vi "Compare.vi"(8 "error in":errorcluster, 10 "Actual":refnum<class "CANopen Response Message.lvclass">, 11 "Initiate Down-Upload Response Comparator in":refnum<class "Initiate Down-Upload Response Comparator.lvclass">) -> (0 "error out":errorcluster, 2 "Equal?":bool, 3 "Initiate Down-Upload Response Comparator out":refnum<class "Initiate Down-Upload Response Comparator.lvclass">)   [LabVIEW 2024, in "CANopen Master.lvlib" / "Initiate Down-Upload Response Comparator.lvclass"]
uses:
  Initiate Down-Upload Response Comparator.lvclass
  D:/git/CANopen-XNET/SDO Response Compare Strategy/SDO Response Compare Strategy.lvclass
  CANopen Response/CANopen Response Message.lvclass
  D:/git/CANopen-XNET/CANopen Message/CANopen Message.lvclass
  SDO Response Compare Strategy/SDO Response Compare Strategy.lvclass/SDO Response Compare Strategy.ctl
  CANopen Message/CANopen Message.lvclass/CANopen Message.ctl
  CANopen Message/CANopen Message.lvclass
  SDO Response Compare Strategy/SDO Response Compare Strategy.lvclass
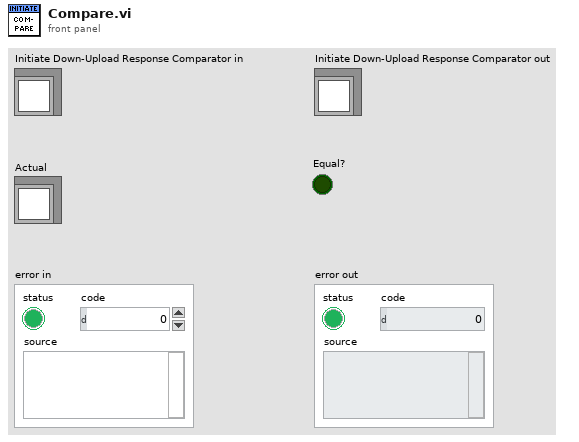
[diagram p1: front panel]
types:
  T1 = typedef "CANopen Master.lvlib/Multiplexor.ctl" = cluster{"Index":u16, "Sub-Index":u8}
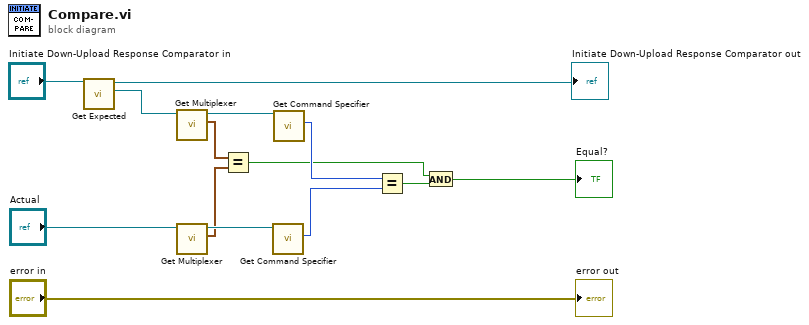
[diagram p0: block diagram]
diagram:
  n1 = call "Get Expected.vi"("SDO Response Compare Strategy in"="Initiate Down-Upload Response Comparator in") -> ("Expected Response Message"=w4:refnum<class "CANopen Response Message.lvclass">, "SDO Response Compare Strategy out"=→"Initiate Down-Upload Response Comparator out":refnum<class "Initiate Down-Upload Response Comparator.lvclass">)  [unwired: 9 in]
  n2 = call "Get Multiplexer.vi"("CANopen Message in"=w4) -> ("Multiplexer"=w9:T1, "CANopen Message out"=w11:refnum<class "CANopen Response Message.lvclass">)  [unwired: 9 in]
  n3 = call "Get Multiplexer.vi"("CANopen Message in"="Actual") -> ("Multiplexer"=w8:T1, "CANopen Message out"=w10:refnum<class "CANopen Response Message.lvclass">)  [unwired: 9 in]
  n4 = Equal?(x=w9, y=w8) -> (x = y?=w7:bool)
  n5 = call "Get Command Specifier.vi"("CANopen Message in"=w10) -> ("Command Specifier"=w13:u8)  [unwired: 9 in, 1 out]
  n6 = call "Get Command Specifier.vi"("CANopen Message in"=w11) -> ("Command Specifier"=w14:u8)  [unwired: 9 in, 1 out]
  n7 = Equal?(x=w14, y=w13) -> (x = y?=w12:bool)
  n8 = And(x=w7, y=w12) -> (x .and. y?=→"Equal?":bool)
  "error out" <- "error in"
